vi "Controller Write FXP20.5.vi"(8 "Error In":errorcluster, 10 "Values":fxp<+/-,20,5>[](array[numeric]), 11 "Variables":refnum<k21>[](array[refnum])) -> (0 "Error Out":errorcluster)   [LabVIEW 2011, in "Controller VIs.lvlib"]
doc: "Writes a vector of fixed-Point <+/-,20,5> I/O variables."
uses:
  Controller VIs.lvlib
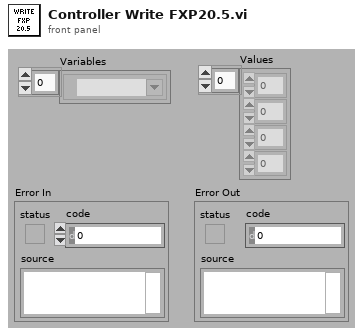
[diagram p1: front panel]
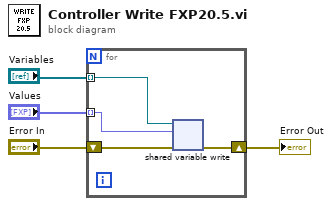
[diagram p0: block diagram]
diagram:
  n1 = for {
    tunnel: "Values" -> [w5] mode=indexing
    tunnel: "Variables" -> [w8] mode=indexing
    shift-right: [w6] -> w3
    shift-left: "Error In" -> [w7]
    n2 = shared-variable-write(w8, w7, w5) -> (w6:errorcluster)  [unwired: 1 out]
  }
  "Error Out" <- w3
